vi "symmetry property2.vi"() -> ()   [LabVIEW 2014]
panel:
  out "Waveform Chart":dbl[][](graph)
  in  "stop 2":bool
  in  "stop":bool
  out "Waveform Chart 2":dbl[][](graph)
  out "OUTPUT- 2":dbl[][](array[numeric]) format="%#.3f"
  in  "N 2":dbl
  out "OUTPUT-1":dbl[][](array[numeric]) format="%#.3f"
  in  "N":dbl
  # "SYMMETRY PROPERTY-2"
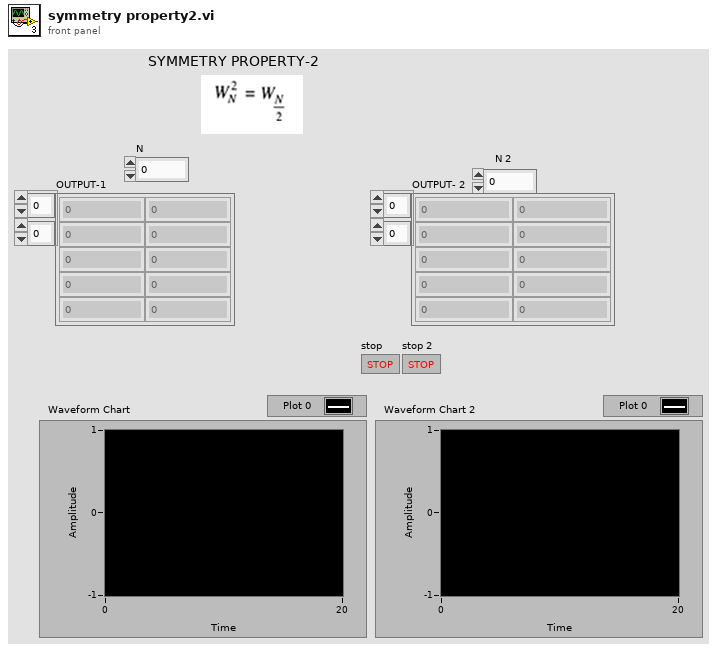
[diagram p1: front panel]
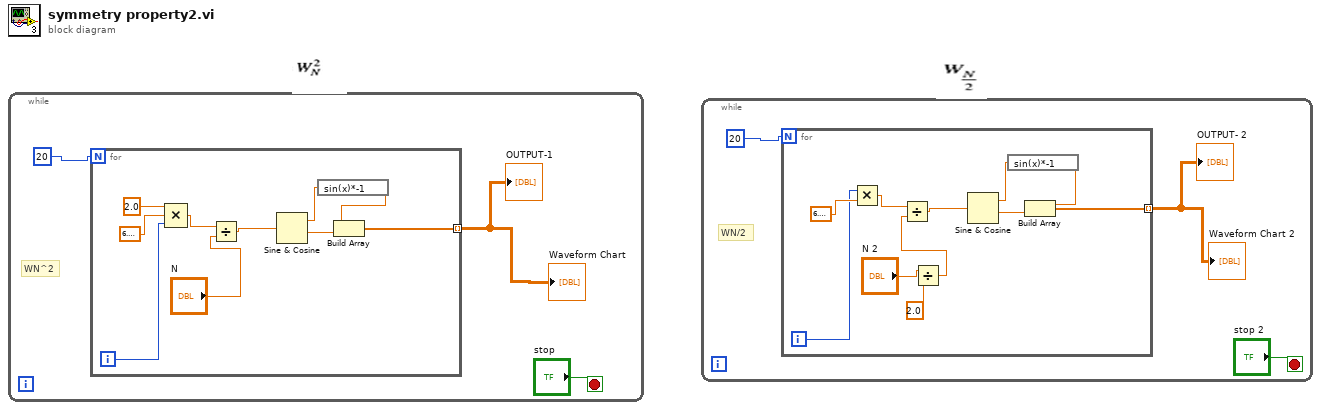
[diagram p0: block diagram]
diagram:
  n1 = while {
    stop <- "stop" stop-if-true
    # "WN^2"
    n2 = for {
      N: 20 -> [_]
      tunnel: [w5] -> w2 mode=indexing
      i -> [w11]
      n3 = Compound Arithmetic op=MULTIPLY(2.0 ("x"), 6.283185307179586, w11) -> (w10:dbl)
      n4 = Divide(x=w10, y="N") -> (x/y=w8:dbl)
      n5 = Sine & Cosine(0:w8) -> (1:w7:dbl, 2:w6:dbl)
      n6 = expression code="sin(x)*-1"(w7) -> (w4:dbl)
      n7 = Build Array(w4, w6) -> (w5:dbl[])
    }
    "OUTPUT-1" <- w2
    "Waveform Chart" <- w2
  }
  n8 = while {
    stop <- "stop 2" stop-if-true
    # "WN/2"
    n9 = for {
      N: 20 -> [_]
      tunnel: [w21] -> w16 mode=indexing
      i -> [w26]
      n10 = Multiply(x=w26, y=6.283185307179586) -> (x*y=w25:dbl)
      n11 = Divide(x="N 2", y=2.0) -> (x/y=w19:dbl)
      n12 = Divide(x=w25, y=w19) -> (x/y=w24:dbl)
      n13 = Sine & Cosine(0:w24) -> (1:w23:dbl, 2:w22:dbl)
      n14 = expression code="sin(x)*-1"(w23) -> (w17:dbl)
      n15 = Build Array(w17, w22) -> (w21:dbl[])
    }
    "OUTPUT- 2" <- w16
    "Waveform Chart 2" <- w16
  }
